vi "Camera.vi"() -> ()   [LabVIEW 2016]
uses:
  <vilib>/rvi/Emulation/niFpgaGetClockAttributes.vi
  <vilib>/rvi/Emulation/niFpgaSctlEmulationGetInTimedLoop.vi
  <vilib>/rvi/Emulation/niFpgaEmulationReportErrorSimple.vi
  <vilib>/rvi/eio/common/nirviEmuTemplateMethod_errors.vi
  <vilib>/rvi/Emulation/niFpgaCriticalErrorInLSC.vi
  <vilib>/eio/EIONode/EIONode.xnode
panel:
  in  "Tlow = t":i16=9
  in  "Fly View Frame Rate = R":i16=10
  in  "Arena View Frame Rate = R":i16=200
  out "Camera flash time":i16
  in  "Camera flash time t":i16
  in  "Camera offset = x":i16=150
  in  "Flash":bool
  # "** Frequency  = 1 / (Fly View R * 0.0001)   \ni.e R = 10, Frequency = 1000Hz"
  # "**T period = R*100µs,      T low = t*100 µs"
  # "** Frequency  = 1 / (R * 0.0001)   \ni.e R = 200, Frequency = 50Hz"
  # "** Trigger the fluorenscence camera (Arena View R - x ) *100 microseconds earlier\n      i.e Arena View R = 200, x = 150,\n           offset x = (200 - 150) * 100 µs = 50 µs"
  # "** Camera flash time is set to be the time for triggering the flash at the end of every video.\n** The unit is second."
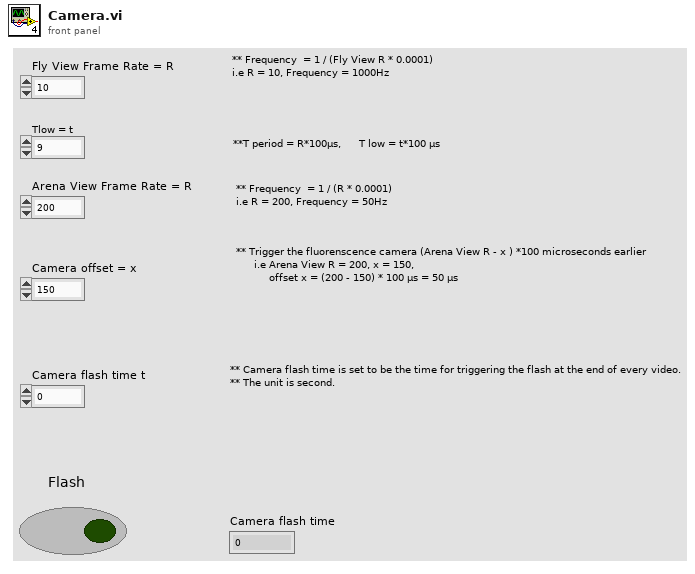
[diagram p1: front panel]
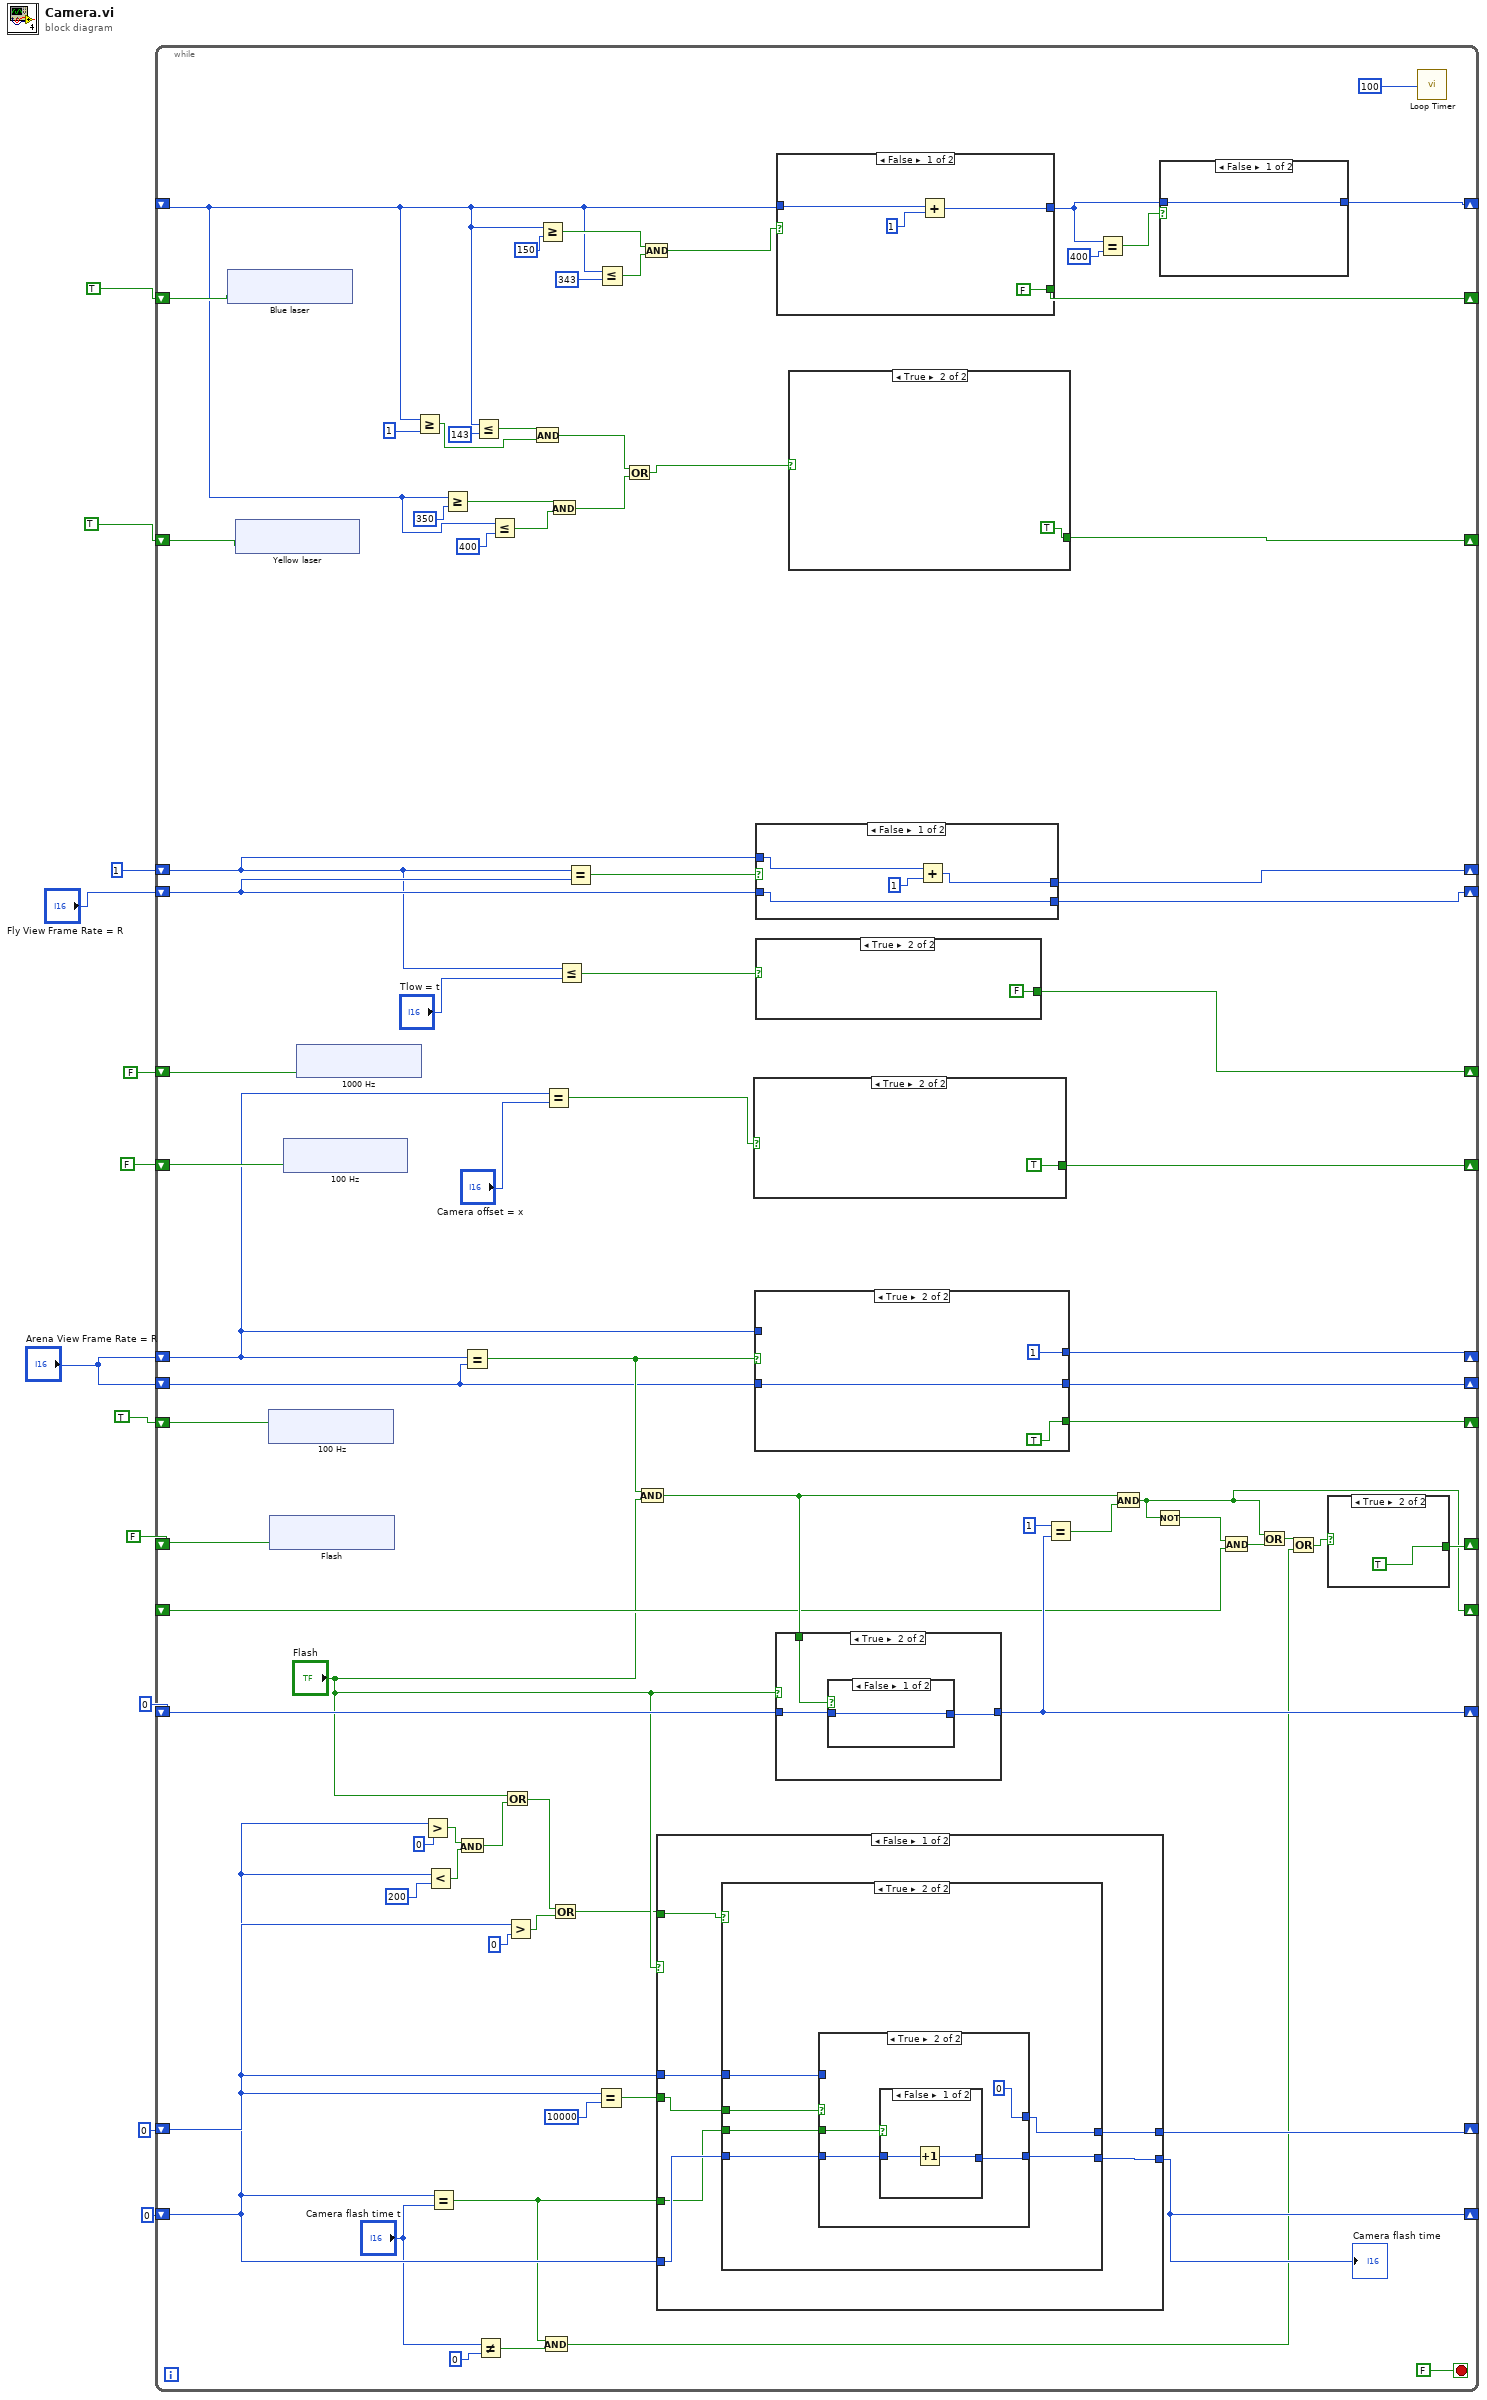
[diagram p0: block diagram]
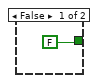
[diagram p2: hidden frame]
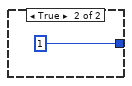
[diagram p3: hidden frame]
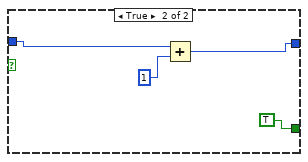
[diagram p4: hidden frame]
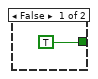
[diagram p5: hidden frame]
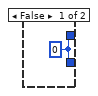
[diagram p6: hidden frame]
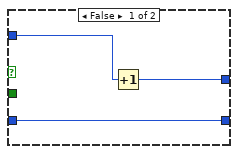
[diagram p7: hidden frame]
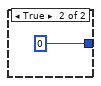
[diagram p8: hidden frame]
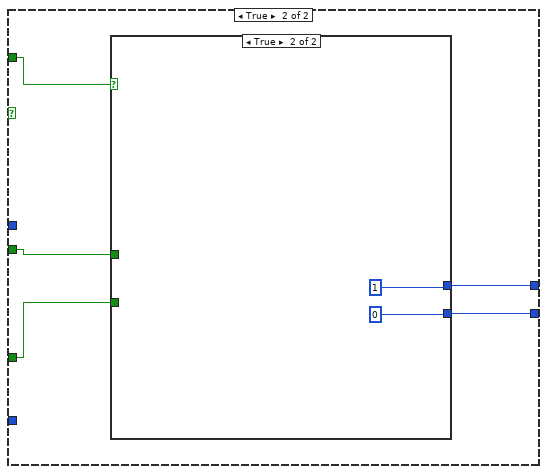
[diagram p9: hidden frame]
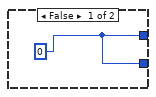
[diagram p10: hidden frame]
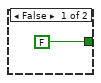
[diagram p11: hidden frame]
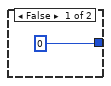
[diagram p12: hidden frame]
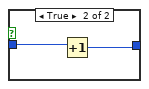
[diagram p13: hidden frame]
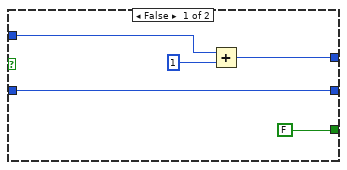
[diagram p14: hidden frame]
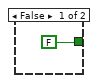
[diagram p15: hidden frame]
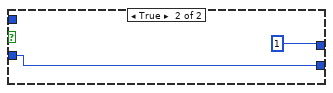
[diagram p16: hidden frame]
diagram:
  n1 = while {
    shift-right: [w42] -> _
    shift-left: FALSE -> [w93]
    shift-right: [w91] -> _
    shift-left: i16 1 -> [w38]
    shift-right: [w88] -> _
    shift-left: FALSE -> [w89]
    shift-right: [w87] -> _
    shift-left: TRUE -> [w82]
    shift-right: [w86] -> _
    shift-left: "Arena View Frame Rate = R" -> [w77]
    shift-right: [w79] -> _
    shift-left: i16 0 -> [w83]
    shift-right: [w75] -> _
    shift-left: FALSE -> [w76]
    shift-right: [w71] -> _
    shift-left: _ -> [w72]
    shift-right: [w64] -> _
    shift-left: i16 0 -> [w57]
    shift-right: [w65] -> _
    shift-left: i16 0 -> [w51]
    shift-right: [w45] -> _
    shift-left: "Arena View Frame Rate = R" -> [w44]
    shift-right: [w43] -> _
    shift-left: "Fly View Frame Rate = R" -> [w41]
    shift-right: [w18] -> _
    shift-left: TRUE -> [w17]
    shift-right: [w16] -> _
    shift-left: TRUE -> [w15]
    shift-right: [w14] -> _
    shift-left: _ -> [w13]
    stop <- FALSE stop-if-true
    n2 = xnode "Blue laser"("ConnectorC/DIO4"=w15) -> ()  [unwired: 1 in, 1 out]
    n3 = xnode "Yellow laser"("ConnectorC/DIO5"=w17) -> ()  [unwired: 1 in, 1 out]
    n4 = xnode "100 Hz"("ConnectorC/DIO2"=w82) -> ()  [unwired: 1 in, 1 out]
    n5 = xnode "Flash"("ConnectorC/DIO3"=w76) -> ()  [unwired: 1 in, 1 out]
    n6 = xnode "100 Hz"("ConnectorC/DIO1"=w89) -> ()  [unwired: 1 in, 1 out]
    n7 = xnode "1000 Hz"("ConnectorC/DIO0"=w93) -> ()  [unwired: 1 in, 1 out]
    n8 = Greater Or Equal?(x=w13, y=i16 1) -> (x >= y?=w31:bool)
    n9 = Greater?(x=w51, y=i16 0) -> (0:w54:bool)
    n10 = Less?(x=w51, y=i16 200) -> (x < y?=w53:bool)
    n11 = Equal?(x=w51, y="Camera flash time t") -> (x = y?=w47:bool)
    n12 = Greater Or Equal?(x=w13, y=i16 350) -> (x >= y?=w28:bool)
    n13 = And(x=w54, y=w53) -> (x .and. y?=w52:bool)
    n14 = Equal?(x=w77, y=w44) -> (x = y?=w84:bool)
    n15 = Less Or Equal?(x=w13, y=i16 143) -> (x <= y?=w30:bool)
    n16 = Not Equal?(x="Camera flash time t", y=i16 0) -> (x != y?=w48:bool)
    n17 = Less Or Equal?(x=w13, y=i16 400) -> (x <= y?=w27:bool)
    n18 = Or(x="Flash", y=w52) -> (x .or. y?=w59:bool)
    n19 = Greater?(x=w57, y=i16 0) -> (0:w60:bool)
    n20 = And(x=w30, y=w31) -> (x .and. y?=w32:bool)
    n21 = Greater Or Equal?(x=w13, y=i16 150) -> (x >= y?=w35:bool)
    n22 = And(x=w47, y=w48) -> (x .and. y?=w46:bool)
    n23 = Equal?(x=w77, y="Camera offset = x") -> (x = y?=w90:bool)
    n24 = And(x=w28, y=w27) -> (x .and. y?=w29:bool)
    n25 = Or(x=w59, y=w60) -> (x .or. y?=w58:bool)
    n26 = Less Or Equal?(x=w38, y="Tlow = t") -> (x <= y?=w40:bool)
    n27 = Equal?(x=w38, y=w41) -> (x = y?=w85:bool)
    n28 = Equal?(x=w57, y=i16 10000) -> (x = y?=w63:bool)
    n29 = Less Or Equal?(x=w13, y=i16 343) -> (x <= y?=w36:bool)
    n30 = Or(x=w32, y=w29) -> (x .or. y?=w22:bool)
    n31 = And(x=w84, y="Flash") -> (x .and. y?=w81:bool)
    n32 = And(x=w35, y=w36) -> (x .and. y?=w37:bool)
    n33 = case shown="False" "Flash" {
      tunnel: [w113 w136] -> w65
      tunnel: [w114 w135] -> w64
      tunnel: w57 -> [w111 _]
      tunnel: w63 -> [w112 w134]
      tunnel: w47 -> [w108 w133]
      tunnel: w51 -> [w110 _]
      tunnel: w58 -> [w109 w132]
      frame False {
        n34 = case shown="True" w109 {
          tunnel: [w115 w119] -> w114
          tunnel: [w115 w118] -> w113
          tunnel: w112 -> [_ w121]
          tunnel: w111 -> [_ w120]
          tunnel: w110 -> [_ w117]
          tunnel: w108 -> [_ w116]
          frame False {
            w115 = i16 0
          }
          frame True {
            n35 = case shown="True" w121 {
              tunnel: w120 -> [w124 _]
              tunnel: [w123 i16 0] -> w119
              tunnel: [w122 w127] -> w118
              tunnel: w117 -> [w122 w126]
              tunnel: w116 -> [_ w125]
              frame False {
                n36 = Increment(x=w124) -> (x+1=w123:i16)
              }
              frame True {
                n37 = case shown="False" w125 {
                  tunnel: [w129 i16 0] -> w127
                  tunnel: w126 -> [w130 _]
                  frame False {
                    n38 = Increment(x=w130) -> (x+1=w129:i16)
                  }
                  frame True {
                  }
                }
              }
            }
          }
        }
      }
      frame True {
        n39 = case shown="True" w132 {
          tunnel: [w137 i16 1] -> w135
          tunnel: w133 -> [_ _]
          tunnel: [w137 i16 0] -> w136
          tunnel: w134 -> [_ _]
          frame False {
            w137 = i16 0
          }
          frame True {
          }
        }
      }
    }
    "Camera flash time" <- w65
    n40 = case shown="True" w90 {
      tunnel: [FALSE TRUE] -> w88
      frame False {
      }
      frame True {
      }
    }
    n41 = case shown="True" w84 {
      tunnel: [FALSE TRUE] -> w87
      tunnel: [w151 i16 1] -> w86
      tunnel: w77 -> [w153 _]
      tunnel: [w149 w154] -> w45
      tunnel: w44 -> [w149 w154]
      frame False {
        n42 = Add(x=w153, y=i16 1) -> (x+y=w151:i16)
      }
      frame True {
      }
    }
    n43 = case shown="True" w40 {
      tunnel: [TRUE FALSE] -> w42
      frame False {
      }
      frame True {
      }
    }
    n44 = case shown="False" w85 {
      tunnel: [w161 i16 1] -> w91
      tunnel: w38 -> [w160 _]
      tunnel: [w159 w163] -> w43
      tunnel: w41 -> [w159 w163]
      frame False {
        n45 = Add(x=w160, y=i16 1) -> (x+y=w161:i16)
      }
      frame True {
      }
    }
    n46 = case shown="True" "Flash" {
      tunnel: w83 -> [_ w144]
      tunnel: [i16 0 w143] -> w79
      tunnel: w81 -> [_ w145]
      frame False {
      }
      frame True {
        n47 = case shown="False" w145 {
          tunnel: w144 -> [w146 w148]
          tunnel: [w146 w147] -> w143
          frame False {
          }
          frame True {
            n48 = Increment(x=w148) -> (x+1=w147:i16)
          }
        }
      }
    }
    n49 = case shown="False" w37 {
      tunnel: w13 -> [w100 w103]
      tunnel: [w99 w102] -> w21
      tunnel: [FALSE TRUE] -> w16
      frame False {
        n50 = Add(x=w100, y=i16 1) -> (x+y=w99:i16)
      }
      frame True {
        n51 = Add(x=w103, y=i16 1) -> (x+y=w102:i16)
      }
    }
    n52 = case shown="True" w22 {
      tunnel: [FALSE TRUE] -> w18
      frame False {
      }
      frame True {
      }
    }
    n53 = Equal?(x=i16 1, y=w79) -> (x = y?=w78:bool)
    n54 = Equal?(x=w21, y=i16 400) -> (x = y?=w20:bool)
    n55 = And(x=w81, y=w78) -> (x .and. y?=w71:bool)
    n56 = Not(x=w71) -> (.not. x?=w73:bool)
    n57 = case shown="False" w20 {
      tunnel: [w96 i16 1] -> w14
      tunnel: w21 -> [w96 _]
      frame False {
      }
      frame True {
      }
    }
    n58 = And(x=w73, y=w72) -> (x .and. y?=w74:bool)
    n59 = Or(x=w71, y=w74) -> (x .or. y?=w68:bool)
    n60 = Or(x=w68, y=w46) -> (x .or. y?=w67:bool)
    n61 = case shown="True" w67 {
      tunnel: [FALSE TRUE] -> w75
      frame False {
      }
      frame True {
      }
    }
    n62 = call "Loop Timer"("Count(uSec)"=u32 100) -> ()  [unwired: 1 out]
  }
